vi "Fehlerauswertung.vi"(10 "Empfangsdaten":string[](array[string])) -> (1 "Error":T1, 2 "Alarme":string)   [LabVIEW 2020, in "Linearisierung v2.lvlib" / "Gasteiler.lvlib" / "AK Komm Gasteiler.lvlib"]
uses:
  AK Komm Gasteiler.lvlib
  Gasteiler Fehler.ctl
  Gasteiler.lvlib
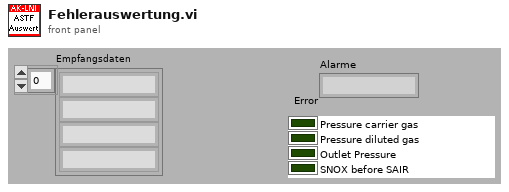
[diagram p1: front panel]
types:
  T1 = typedef "Linearisierung v2.lvlib/Gasteiler.lvlib/Gasteiler Fehler.ctl" = cluster{"Pressure carrier gas":bool, "Pressure diluted gas":bool, "Outlet Pressure":bool, "SNOX before SAIR":bool}
  T2 = cluster{"Error[0]":bool, "Error[1]":bool, "Error[2]":bool, "Error[3]":bool}
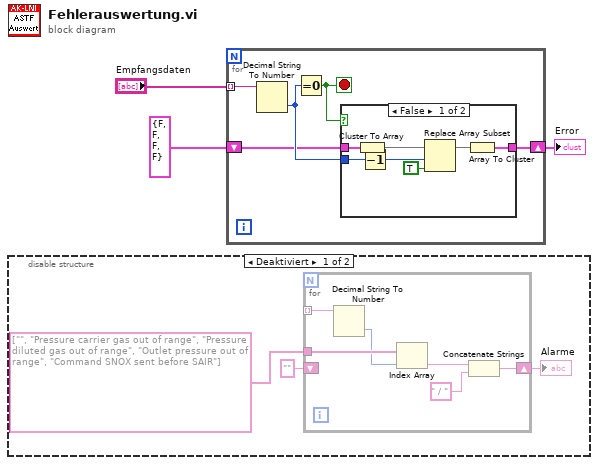
[diagram p0: block diagram]
diagram:
  n1 = disable-structure shown="Deaktiviert" {
    frame Disabled {
      n2 = for {
        tunnel: [w13] -> w7 mode=indexing
        tunnel: string[] ["", "Pressure carrier gas out of range", "Pressure diluted gas out of range", "Outlet pressure out of range", "Command SNOX sent before SAIR"] ("Empfangsdaten") -> [w12]
        shift-right: [w8] -> w4
        shift-left: "" -> [_]
        n3 = Decimal String To Number(string=w13) -> (number=w11:i32)  [unwired: 2 in, 1 out]
        n4 = Index Array(array=w12, index=w11) -> (element=w10:string)
        n5 = Concatenate Strings(w10, " / " ("String")) -> (w8:string)
      }
      "Alarme" <- w4
    }
    frame Enabled {
    }
  }
  n6 = for {
    tunnel: "Empfangsdaten" -> [w18] mode=indexing
    shift-right: [w14] -> w1
    shift-left: T1 {"Pressure carrier gas"=FALSE, "Pressure diluted gas"=FALSE, "Outlet Pressure"=FALSE, "SNOX before SAIR"=FALSE} ("Error") -> [w15]
    stop <- w16 stop-if-true
    n7 = Decimal String To Number(string=w18) -> (number=w17:i32)  [unwired: 2 in, 1 out]
    n8 = Equal To 0?(x=w17) -> (x = 0?=w16:bool)
    n9 = case shown="False" w16 {
      tunnel: w17 -> [w25 _]
      tunnel: w15 -> [w23 w26]
      tunnel: [w19 w26] -> w14
      frame False {
        n10 = Cluster To Array(cluster=w23) -> (array=w22:bool[])
        n11 = Decrement(x=w25) -> (x-1=w24:i32)
        n12 = Replace Array Subset(array=w22, new element=TRUE ("Neues Element/Teil-Array"), index=w24) -> (w20:bool[])
        n13 = Array To Cluster(array=w20) -> (cluster=w19:T2)
      }
      frame True {
      }
    }
  }
  "Error" <- w1
